vi "MainIteratesTempForResonance.vi"() -> ()   [LabVIEW 2010]
panel:
  out "error out":errorcluster
  in  "error in":errorcluster
  in  "#Measurements each Frequency":i32=200
  in  "Step":dbl=200.0 format="%.2f"
  in  "Start":dbl=200.0 format="%.2f"
  in  "Stop":dbl=200.0 format="%.2f"
  in  "Voltage Stop":dbl=200.0 format="%.2f"
  in  "Voltage Step":dbl=200.0 format="%.2f"
  in  "Voltage Start":dbl=200.0 format="%.2f"
  in  "Wait equilibrium (min)":dbl=200.0 format="%.2f"
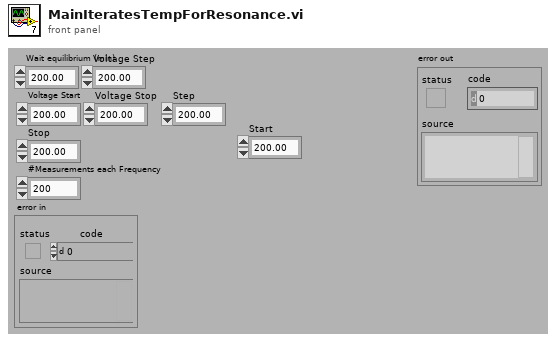
[diagram p1: front panel]
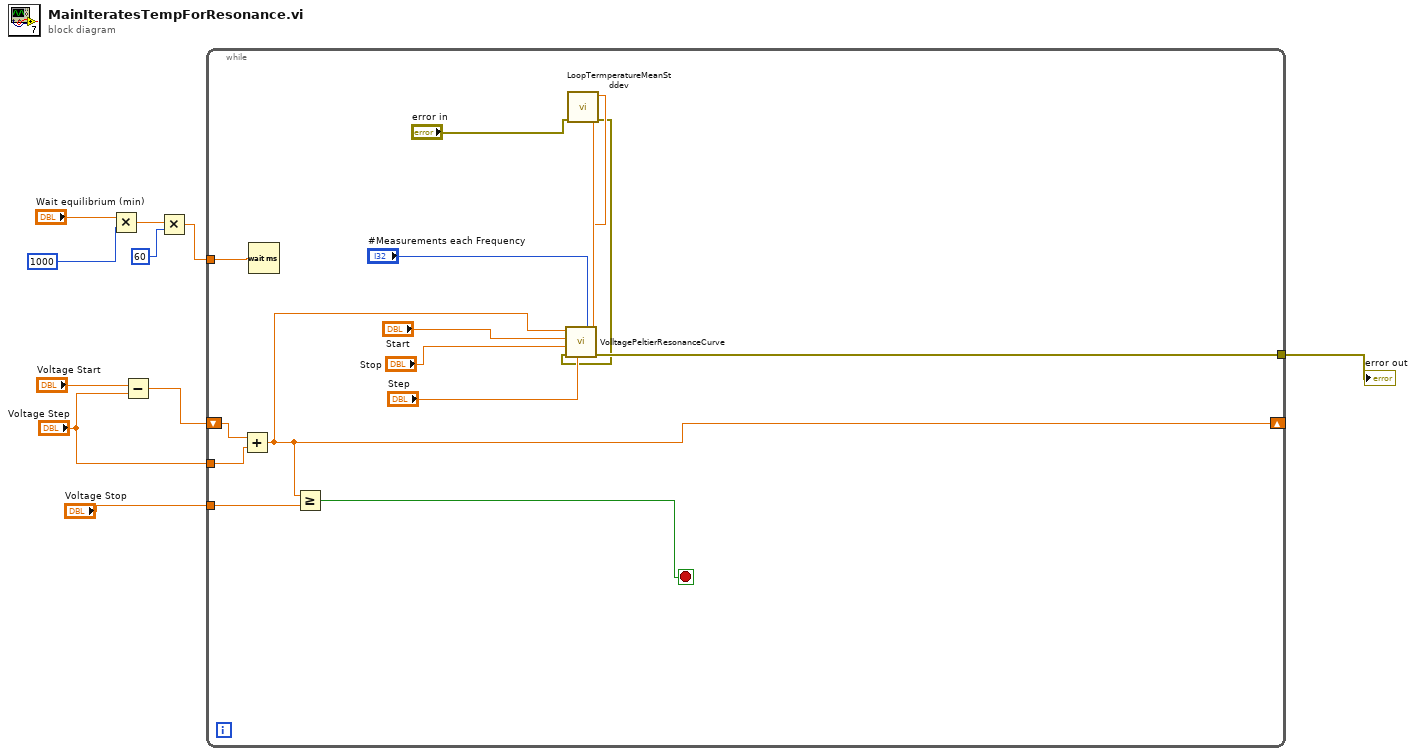
[diagram p0: block diagram]
diagram:
  n1 = Multiply(x="Wait equilibrium (min)", y=1000) -> (x*y=w8:dbl)
  n2 = Subtract(x="Voltage Start", y="Voltage Step") -> (x-y=w4:dbl)
  n3 = Multiply(x=w8, y=60) -> (x*y=w6:dbl)
  n4 = while {
    tunnel: w6 -> [w25]
    shift-right: [w16] -> _
    shift-left: w4 -> [w23]
    tunnel: "Voltage Step" -> [w24]
    tunnel: "Voltage Stop" -> [w22]
    tunnel: [w20] -> w1
    stop <- w21 stop-if-true
    n5 = Add(x=w23, y=w24) -> (x+y=w16:dbl)
    n6 = Wait (ms)(milliseconds to wait=w25) -> ()  [unwired: 1 out]
    n7 = Greater Or Equal?(x=w16, y=w22) -> (x >= y?=w21:bool)
    n8 = call "LoopTermperatureMeanStddev.vi"("error in 2"="error in") -> ("error out 2"=w11:errorcluster, "Temperature Error"=w14:dbl, "Temperature"=w13:dbl)  [unwired: 8 in]
    n9 = call "VolltagePeltierResonanceCurve.vi"("TemperatureError"=w14, "Temperature"=w13, "#Measurements each Frequency"="#Measurements each Frequency", "Step"="Step", "error in"=w11, "Stop"="Stop", "Start"="Start", "Voltage"=w16) -> ("error out"=w20:errorcluster)  [unwired: 3 in]
  }
  "error out" <- w1
